vi "AddNewSlideIntoListing.vi"(1 "Old Listing":string[][](array[string]), 2 "name":string) -> (0 "New listing":string[][](array[string]))   [LabVIEW 2014]
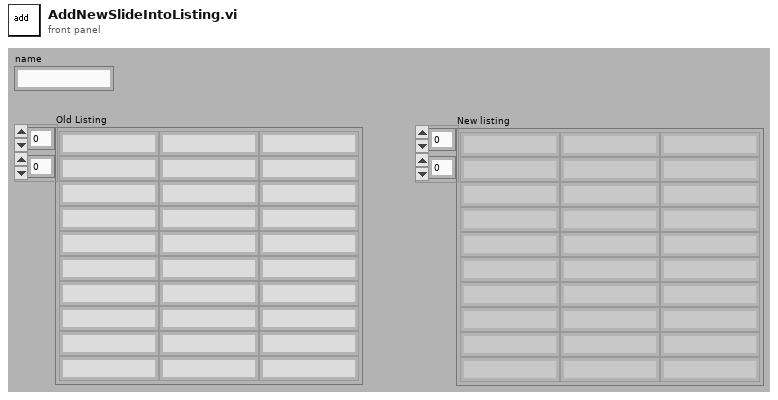
[diagram p1: front panel]
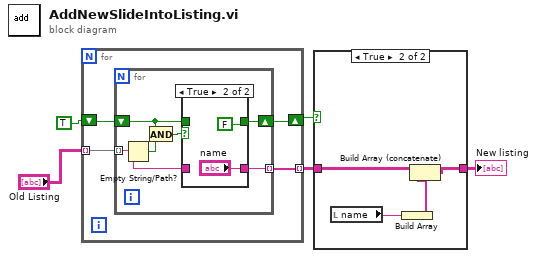
[diagram p0: block diagram]
diagram:
  n1 = for {
    tunnel: "Old Listing" -> [w9] mode=indexing
    shift-right: [w7] -> w3
    shift-left: TRUE -> [w8]
    tunnel: [w6] -> w1 mode=indexing
    n2 = for {
      tunnel: w9 -> [w12] mode=indexing
      shift-right: [w11] -> w7
      shift-left: w8 -> [w10]
      tunnel: [w13] -> w6 mode=indexing
      n3 = Empty String/Path?(string/path=w12) -> (empty?=w14:bool)
      n4 = And(x=w10, y=w14) -> (x .and. y?=w15:bool)
      n5 = case shown="True" w15 {
        tunnel: [w17 "name"] -> w13
        tunnel: w12 -> [w17 _]
        tunnel: [w16 FALSE] -> w11
        tunnel: w10 -> [w16 _]
        frame False {
        }
        frame True {
        }
      }
    }
  }
  n6 = case shown="True" w3 {
    tunnel: [w20 w23] -> w2
    tunnel: w1 -> [w20 w24]
    frame False {
    }
    frame True {
      n7 = local read "name"() -> (w22:string)
      n8 = Build Array(w22) -> (w21:string[])
      n9 = Build Array (concatenate)(w24, w21) -> (w23:string[][])
    }
  }
  "New listing" <- w2
